vi "Set Device Parameters.vi"(8 "error in":errorcluster, 10 "device parameters":T1={"initialization method"=enum."PXI Slot Number", "card number"=0, "PXI slot number"=2, "core number"=0}, 11 "Ballard MIL-STD 1553 custom device in":T3=18446744073709551615 format="%.0x") -> (0 "error out":errorcluster, 3 "Ballard MIL-STD 1553 custom device out":T3 format="%.0x")   [LabVIEW 2020, in "Ballard MIL-STD-1553 Scripting.lvlib"]
doc: "Specifies Ballard hardware device parameters such as <b>PXI slot number</b> and <b>core number</b>."
uses:
  Ballard MIL-STD-1553 Scripting.lvlib
  <vilib>/NI VeriStand/Custom Device API/Custom Device Item Ref.ctl
  Shared/Device Parameters.ctl
  Shared/Initialization Method.ctl
  Constants.vi
  <vilib>/NI VeriStand/Custom Device API/Set Item Property (U16).vi
  <vilib>/NI VeriStand/Custom Device API/Set Item Property (I32).vi
  <vilib>/NI VeriStand/Custom Device API/Custom Device API.lvlib
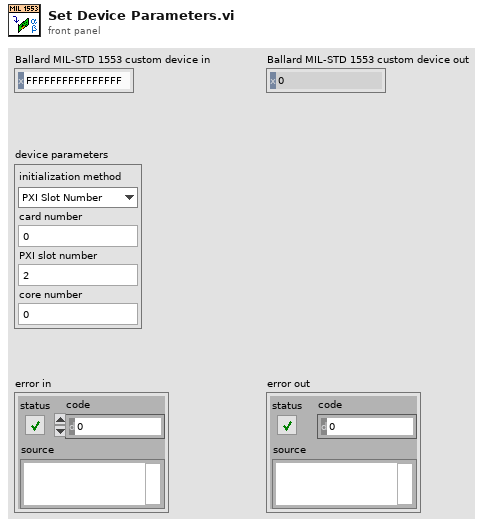
[diagram p1: front panel]
types:
  T1 = typedef "Device Parameters.ctl" = cluster{"initialization method":T2, "card number":i32, "PXI slot number":i32, "core number":i32}
  T2 = typedef "Initialization Method.ctl" = enum16{"PXI Slot Number", "Card Number"}
  T3 = typedef "Custom Device API.lvlib/Custom Device Item Ref.ctl" = u64
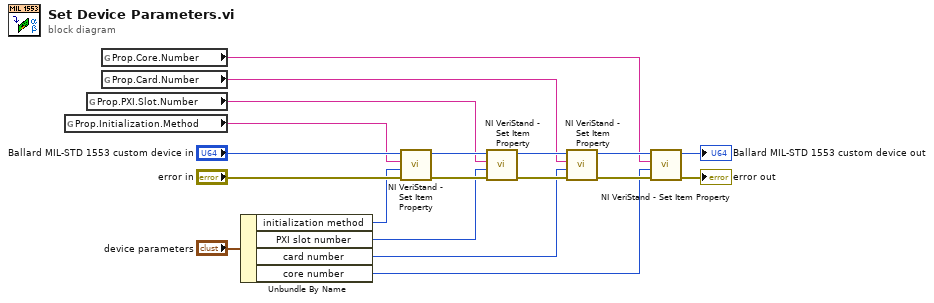
[diagram p0: block diagram]
diagram:
  n1 = global read "Constants.vi" "Prop.Initialization.Method"() -> (w5:string)
  n2 = global read "Constants.vi" "Prop.PXI.Slot.Number"() -> (w4:string)
  n3 = global read "Constants.vi" "Prop.Core.Number"() -> (w2:string)
  n4 = global read "Constants.vi" "Prop.Card.Number"() -> (w3:string)
  n5 = Unbundle By Name("device parameters") -> ("initialization method"=w9:T2, "PXI slot number"=w8:i32, "card number"=w7:i32, "core number"=w6:i32)
  n6 = call-poly <vilib>:"NI VeriStand - Set Item Property.vi"("error in (no error)"="error in", "Value"=w9, "Property Name"=w5, "Item Ref in"="Ballard MIL-STD 1553 custom device in") -> ("error out"=w13:errorcluster, "Item Ref out"=w12:T3)  [unwired: 5 in, 1 out]
  n7 = call-poly <vilib>:"NI VeriStand - Set Item Property.vi"("error in (no error)"=w13, "Value"=w8, "Property Name"=w4, "Item Ref in"=w12) -> ("error out"=w18:errorcluster, "Item Ref out"=w19:T3)  [unwired: 5 in, 1 out]
  n8 = call-poly <vilib>:"NI VeriStand - Set Item Property.vi"("error in (no error)"=w18, "Value"=w7, "Property Name"=w3, "Item Ref in"=w19) -> ("error out"=w16:errorcluster, "Item Ref out"=w17:T3)  [unwired: 5 in, 1 out]
  n9 = call-poly <vilib>:"NI VeriStand - Set Item Property.vi"("error in (no error)"=w16, "Value"=w6, "Property Name"=w2, "Item Ref in"=w17) -> ("error out"=→"error out":errorcluster, "Item Ref out"=→"Ballard MIL-STD 1553 custom device out":T3)  [unwired: 5 in, 1 out]
